vi "PRACTICA 1 DIGITOS BINARIOS Y TEOREMA DE PITAGORAS.vi"() -> ()   [LabVIEW 2017]
panel:
  out "CATETO A":dbl
  out "CATETO B":dbl
  out "C: HIPOTENUSA":dbl
  in  "Lado B":dbl
  in  "Lado A":dbl
  out "Resultado":dbl
  in  "?":bool[](array[boolean])
  # "DIGITOS BINARIOS"
  # "A"
  # "B"
  # "C"
  # "D"
  # "2^2"
  # "2^1"
  # "2^4"
  # "2^0"
  # "TEOREMA DE PITAGORAS"
  # "C"
  # "A"
  # "SALIDA"
  # "B"
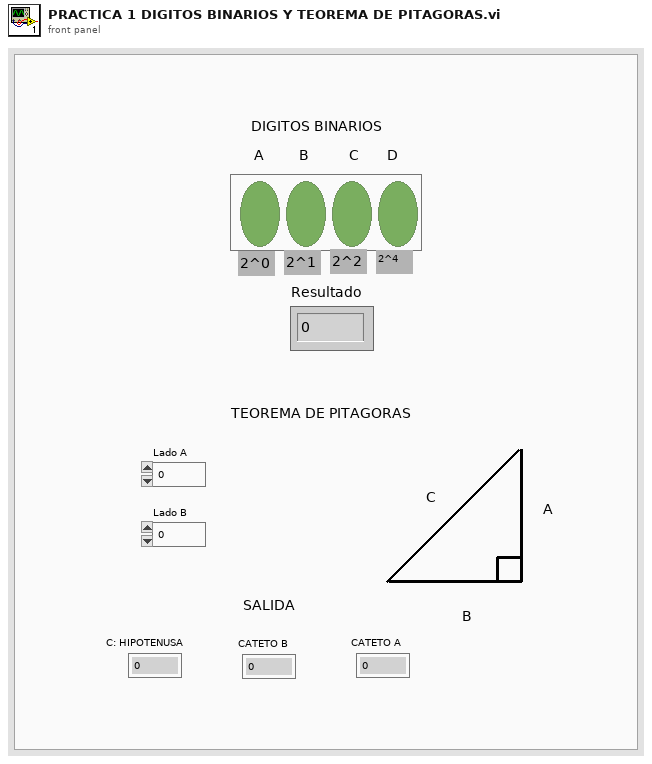
[diagram p1: front panel]
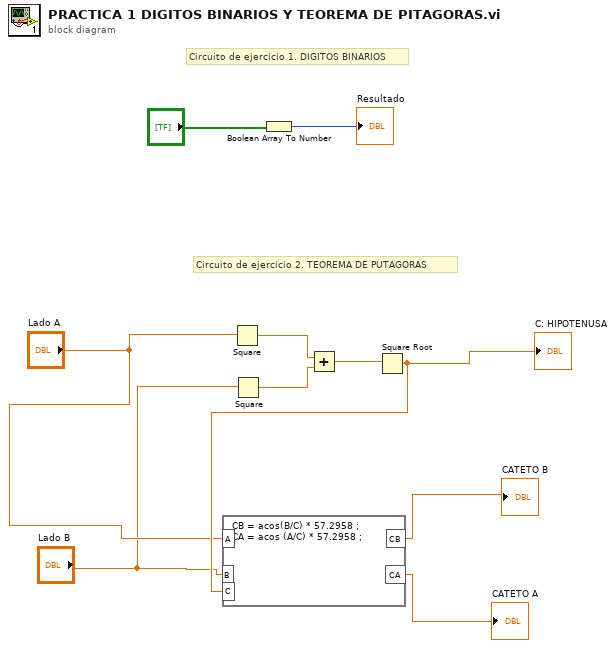
[diagram p0: block diagram]
diagram:
  # "Circuito de ejercicio 2. TEOREMA DE PUTAGORAS"
  # "Circuito de ejercicio 1. DIGITOS BINARIOS"
  n1 = Square(x="Lado A") -> (x^2=w6:dbl)
  n2 = Square(x="Lado B") -> (x^2=w7:dbl)
  n3 = Boolean Array To Number(Boolean array="?") -> (number=→"Resultado":u32)
  n4 = Add(x=w6, y=w7) -> (x+y=w8:dbl)
  n5 = Square Root(x=w8) -> (sqrt(x)=w3:dbl)
  "C: HIPOTENUSA" <- w3
  n6 = formula code="CB = acos(B/C) * 57.2958 ;\nCA = acos (A/C) * 57.2958 ;"("A"="Lado A", "B"="Lado B", "C"=w3) -> ("CB"=→"CATETO B":dbl, "CA"=→"CATETO A":dbl)
